vi "_editDialog.vi"(0 "reference":refnum<class "FinalStateNode.lvclass">, 1 "insidePackageNode":bool, 5 "error in (no error)":errorcluster) -> (14 "reference out":refnum<class "FinalStateNode.lvclass">, 15 "changeConnection":T1, 16 "cancel":bool, 19 "error out":errorcluster)   [LabVIEW 2014, in "FinalStateNode.lvclass"]
doc: "Edit Dialog"
uses:
  <resource>/Framework/Providers/Open_GDS/UML/FinalStateNode_class/FinalStateNode.lvclass
  <resource>/Framework/Providers/Open_GDS/UML/AbstractNode_class/private/NodeConnectionStatsType.ctl
  <resource>/Framework/Providers/Open_GDS/UML/ContextHelp/ContextHelp_HelpTexts.ctl
  <resource>/Framework/Providers/Open_GDS/UML/MultiLineString_class/MultiLineString.lvclass
  <resource>/Framework/Providers/Open_GDS/UML/AbstractNode_class/AbstractNode.lvclass
panel:
  in  "OK Button":bool
  in  "Cancel Button":bool
  in  "Help":bool
  in  "connection":bool caption="Connect to System"
  in  "Initial text":string
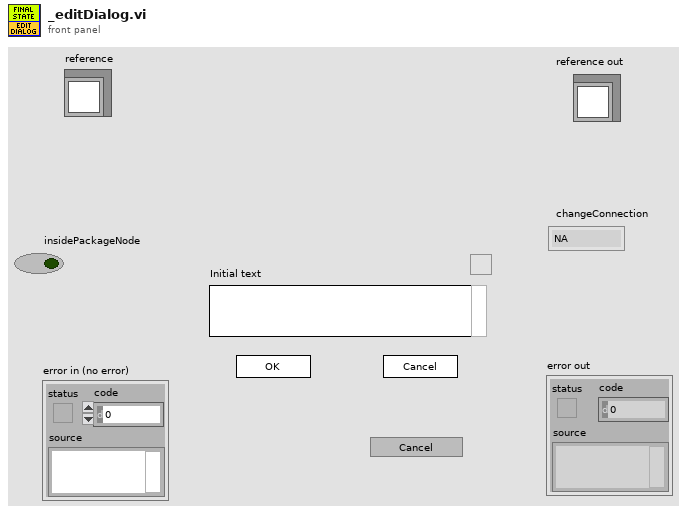
[diagram p1: front panel]
types:
  T1 = typedef "AbstractNode.lvclass/NodeConnectionStatsType.ctl" = enum16{"NA", "Connect", "DisConnect"}
  T2 = typedef "ContextHelp_HelpTexts.ctl" = enum16{"None(Hide)", "Default", "Help", "Welcome", "GettingStarted", "ClassDiagram_Help", "SequenceDiagram_Help", "UseCaseDiagram_Help", "BSelect", "BClass", "BInterface", "BPackage", "BNote", "BDependency", "BInheritance", "BInterfaceImplementation", "BAssociation", "BAggregation", "BCompAggregation", "BNoteConnector", "BObject", "BActionBar", "BCall", "BSystem", "BActor", "BUseCase", "BGeneralization", "BIncludes", "BExtends", "BUseCaseDiagramAssociation", "ClassRelationshipEdge editDialog_Bent Style", "ClassRelationshipEdge editDialog_RelationType", "ClassRelationshipEdge editDialog_Reverse association", "ClassRelationshipEdge editDialog_Start label", "ClassRelationshipEdge editDialog_Middle label", "ClassRelationshipEdge editDialog_End label", "UMLEditor reversedEngineering_Pathes", "ReversedEngineering StateReverseDialog_Help", "ReversedEngineering StateQueuedSettings_Help", "UMLEditor reversedEngineering_AddTopVIs", "UMLEditor reversedEngineering_AddClasses", "UMLEditor reversedEngineering_AddDirs", "UMLEditor reversedEngineering_Recursively", "UMLEditor reversedEngineering_Remove", "UMLEditor reversedEngineering_ClearList", "UMLEditor reversedEngineering_HideSubAss", "UMLEditor reversedEngineering_CreateTypes", "UMLEditor reversedEngineering_OnlyInheritance", "UMLEditor reversedEngineering_CreateApplication", "UMLEditor reversedEngineering_OK", "UMLEditor reversedEngineering_Cancel", "UMLEditor reversedEngineering_Help", "UMLEditor createWizardScriptFile_ScriptfilePath", "UMLEditor createWizardScriptFile_ClassPath", "UMLEditor createWizardScriptFile_Use", "UMLEditor createWizardScriptFile_PrivateDirName", "UMLEditor createWizardScriptFile_DirAppend", "UMLEditor createWizardScriptFile_Separator Character", "UMLEditor createWizardScriptFile_OK", "UMLEditor createWizardScriptFile_Cancel", "UMLEditor createWizardScriptFile_Help", "ClassNode editDialog_Class Name", "InterfaceNode editDialog_Class Name", "ClassNode editDialog_Attribute", "ClassNode editDialog_Methods", "InterfaceNode editDialog_Methods", "ClassNode editDialog_connection", "InterfaceNode editDialog_connection", "ClassNode editDialog_StereoType", "ClassNode editDialog_ShowAttrib", "ClassNode editDialog_ShowMethods", "ClassNode editDialog_ClassPath", "ClassNode editDialog_AddAttribute", "ClassNode editDialog_AddMethod", "InterfaceNode editDialog_AddMethod", "ClassNode AttributeGuide_AttributeName", "ClassNode AttributeGuide_Array?", "ClassNode AttributeGuide_Data Type", "ClassNode AttributeGuide_RefName", "ClassNode AttributeGuide_Preview", "ClassNode AttributeGuide_OK", "ClassNode AttributeGuide_Cancel", "ClassNode MethodGuide_Visibility", "ClassNode MethodGuide_Method Name", "ClassNode MethodGuide_Preview", "ClassNode MethodGuide_OK", "ClassNode MethodGuide_Cancel", "CallNode EditCallProperties_AllButtons", "ObjectNode EditObjectlProperties_AllButtons", "ActorNode EditActorProperties_AllButtons", "UseCaseRelationshipNode EditUseCaselProperties_AllButtons", "UseCaseNode EditUseCaselProperties_AllButtons", "SystemNode EditSystemProperties_AllButtons", "ReversedEngineering UpdateAttributes_AllButtons", "StateNode editDialog_AllButtons", "StateTransition editDialog_AllButtons", "ArrangeNodes Main_Picture", "ArrangeNodes Main_Zoom", "ArrangeNodes Main_Auto Zoom", "ArrangeNodes Main_shorten", "ArrangeNodes Main_Min Length", "ArrangeNodes Main_Max Length", "ArrangeNodes Main_increase", "ArrangeNodes Main_decrease", "ArrangeNodes Main_Shake", "ArrangeNodes Main", "BState", "BInitialState", "BFinalState", "BStateTransition", "StateDiagram_Help", "StateDiagram_PropertiesAllButtons", "ReversedEngineering StateReverseDialog_ClearStates", "ReversedEngineering StateReverseDialog_UseQueuedStateMachines", "ReversedEngineering StateReverseDialog_QueuedSettings", "ReversedEngineering StateReverseDialog_SearchForVIs", "ReversedEngineering StateReverseDialog_SearchCriteria", "OptionsDialog_ClassBasePath", "OptionsDialog_VIPath", "OptionsDialog_ApplicationPath", "OptionsDialog_WizDir", "OptionsDialog_IniFilePath", "OptionsDialog_DefineColors", "OptionsDialog_Help", "OptionsDialog_CreateTypes", "ClassRelationshipEdge editDialog_SplitWire"}
  T3 = typedef "FinalStateNode.lvclass/ObjectAttributes.ctl" = cluster{"name":refnum<class "MultiLineString.lvclass">, "DEFAULT_WIDTH":i32, "DEFAULT_HEIGHT":i32}
  T4 = typedef "AbstractNode.lvclass/ObjectAttributes.ctl" = cluster{"parent":refnum<class "AbstractNode.lvclass">, "children":refnum<class "AbstractNode.lvclass">[], "Hidden":bool}
  T5 = typedef "ContextHelp_ShowType.ctl" = cluster{"Header":string, "Picture":picture, "Text":string}
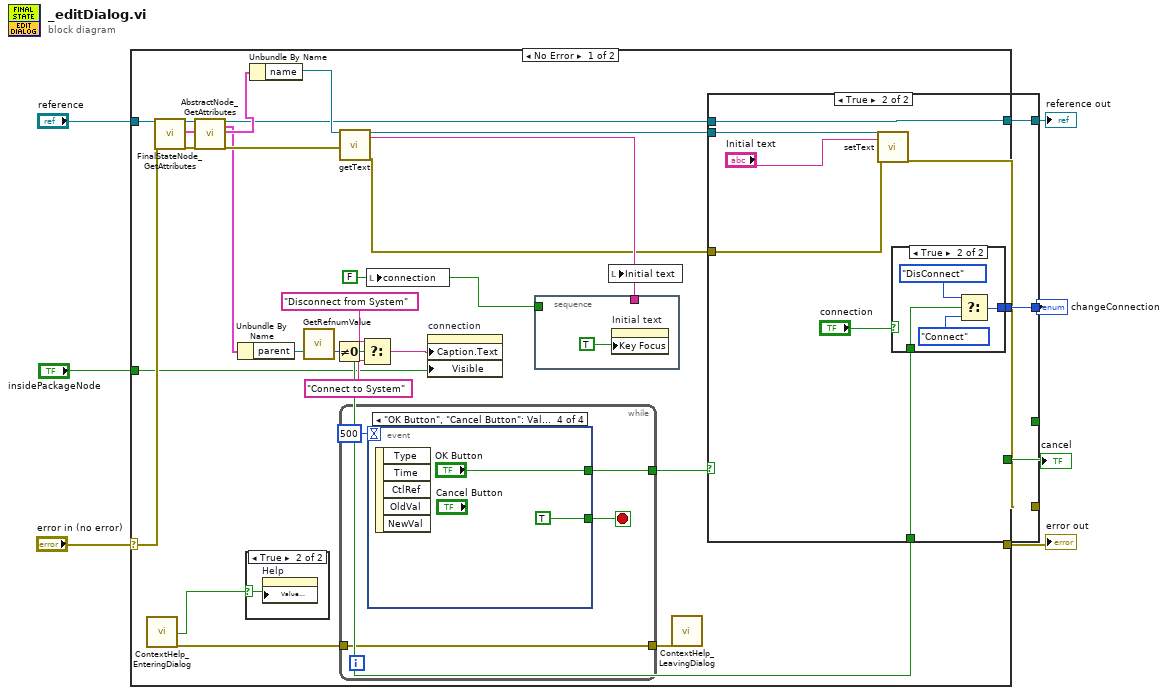
[diagram p0: block diagram]
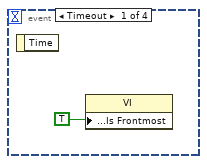
[diagram p3: hidden frame]
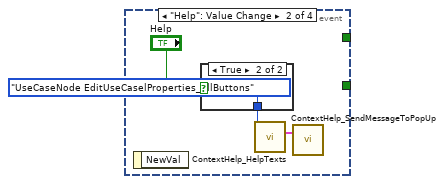
[diagram p4: hidden frame]
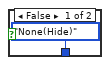
[diagram p5: hidden frame]
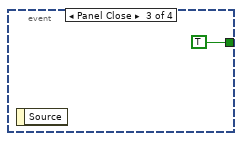
[diagram p6: hidden frame]
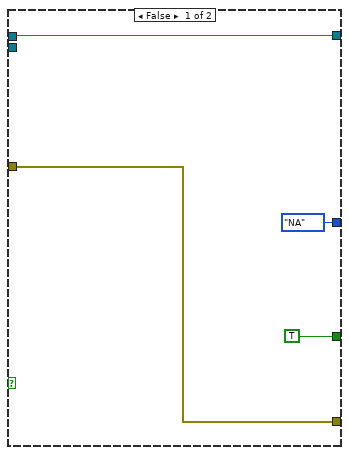
[diagram p7: hidden frame]
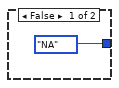
[diagram p8: hidden frame]
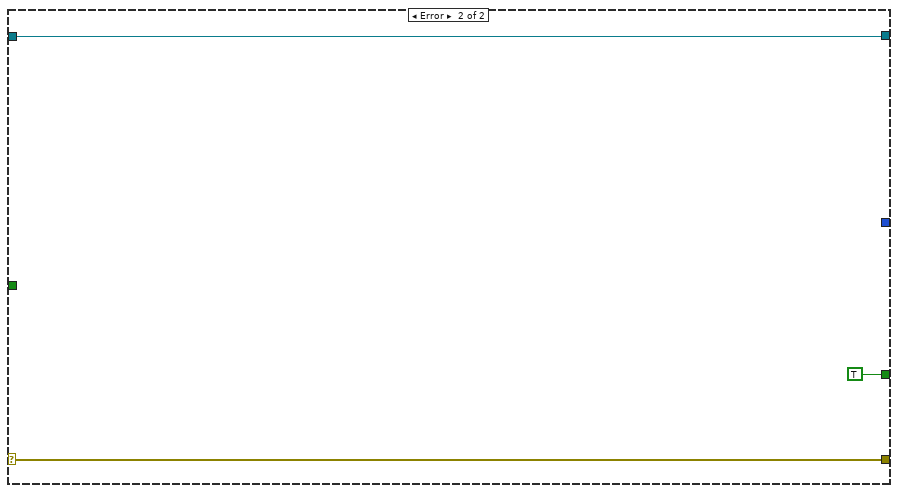
[diagram p9: hidden frame]
diagram:
  n1 = case shown="No Error" "error in (no error)" {
    selector: "error in (no error)" -> [w32 w69]
    tunnel: "reference" -> [w33 w70]
    tunnel: [w35 w69] -> w5
    tunnel: [w34 w70] -> w4
    tunnel: [w28 _] -> w3
    tunnel: "insidePackageNode" -> [w23 _]
    tunnel: [w21 TRUE ("Key Focus")] -> w1
    frame No Error {
      w22 = FALSE ("connection")
      n2 = call <resource>:"ContextHelp_EnteringDialog.vi"() -> ("HelpStatus"=w16:bool, "error out"=w18:errorcluster)  [unwired: 3 in, 15 out]
      n3 = call <resource>:"FinalStateNode_GetAttributes.vi"("reference in"=w33, "error in (no error)"=w32) -> ("reference out"=w12:refnum<class "FinalStateNode.lvclass">, "Data"=w13:T3, "error out"=w11:errorcluster)  [unwired: 1 in, 14 out]
      n4 = call <resource>:"AbstractNode_GetAttributes.vi"("reference in"=w12, "error in (no error)"=w11) -> ("reference out"=w9:refnum<class "FinalStateNode.lvclass">, "Data"=w8:T4, "error out"=w10:errorcluster)  [unwired: 14 in, 1 out]
      n5 = Unbundle By Name(w8) -> ("parent"=w15:refnum<class "AbstractNode.lvclass">)
      n6 = case shown="True" w16 {
        selector: w16 -> [_ w36]
        frame False {
        }
        frame True {
          n7 = property on="Help" class="Bool (strict)"("Value (Signaling)"=w36) -> ()  [unwired: 2 in, 2 out]
        }
      }
      n8 = Unbundle By Name(w13) -> ("name"=w29:refnum<class "MultiLineString.lvclass">)
      n9 = call <resource>:"GetRefnumValue.vi"("reference"=w15) -> ("RefNum"=w14:i32)  [unwired: 17 in, 1 out]
      n10 = Not Equal To 0?(x=w14) -> (x != 0?=w27:bool)
      n11 = call-dynamic "getText.vi"("reference"=w29, "error in (no error)"=w10) -> ("reference out"=w31:refnum<class "MultiLineString.lvclass">, "text"=w30:string, "error out"=w20:errorcluster)  [unwired: 15 in]
      n12 = while {
        tunnel: [w40] -> w17
        tunnel: [w38] -> w19
        tunnel: w18 -> [w38]
        stop <- w39 stop-if-true
        n13 = event shown="[3] \"OK Button\", \"Cancel Button\": Value Change" {
          selector: _ -> [_ _ _ _]
          dyn-events: _ -> [_ _ _ _]
          timeout: 500 -> [_ _ _ _]
          tunnel: [_ _ _ "OK Button"] -> w40
          tunnel: [_ _ TRUE TRUE] -> w39
          event Timeout {
            n14 = event-data() -> ()  [unwired: 2 out]
            n15 = property class="VI"("Front Panel Window:Is Frontmost"=TRUE) -> ()  [unwired: 2 in, 2 out]
          }
          event "Help": Value Change {
            n16 = event-data() -> ()  [unwired: 2 out]
            n17 = case shown="True" "Help" {
              tunnel: [ContextHelp_HelpTexts."None(Hide)" ("HelpText") ContextHelp_HelpTexts."UseCaseNode EditUseCaselProperties_AllButtons" ("HelpText")] -> w43
              frame False {
              }
              frame True {
              }
            }
            n18 = call <resource>:"ContextHelp_HelpTexts.vi"("HelpText (enum or string)"=w43) -> ("HelpOut"=w44:T5)  [unwired: 18 out]
            n19 = call <resource>:"ContextHelp_SendMessageToPopUp.vi"("PopUpMessage"=w44) -> ()  [unwired: 2 in, 17 out]
          }
          event Panel Close {
            n20 = event-data() -> ()  [unwired: 2 out]
          }
          event "OK Button", "Cancel Button": Value Change {
            n21 = event-data() -> ()  [unwired: 6 out]
          }
        }
      }
      n22 = Select(t="Disconnect from System", s=w27, f="Connect to System") -> (s? t:f=w26:string)
      n23 = local write "connection"(w22) -> ()
      n24 = property on="connection" class="Bool (strict)"("Caption.Text"=w26, "Visible"=w23) -> ()  [unwired: 2 in, 2 out]
      n25 = stacked-sequence {
        tunnel: w30 -> [_]
        tunnel: w22 -> [_]
        frame #0 {
          n26 = property on="Initial text" class="Str"("Key Focus"=TRUE) -> ()  [unwired: 2 in, 2 out]
        }
      }
      n27 = local write "Initial text"(w30) -> ()
      n28 = call <resource>:"ContextHelp_LeavingDialog.vi"("error in (no error)"=w19) -> ()  [unwired: 2 in, 17 out]
      n29 = case shown="True" w17 {
        tunnel: [w52 w58] -> w35
        tunnel: [w53 w59] -> w34
        tunnel: w9 -> [w53 w59]
        tunnel: w31 -> [_ w61]
        tunnel: w20 -> [w52 w54]
        tunnel: [enum16{"NA", "Connect", "DisConnect"}."NA" ("changeConnection") w56] -> w28
        tunnel: w27 -> [_ w55]
        tunnel: [TRUE ("Key Focus") _] -> w21
        frame False {
        }
        frame True {
          n30 = call-dynamic "setText.vi"("reference"=w61, "text"="Initial text", "error in (no error)"=w54) -> ("error out"=w58:errorcluster)  [unwired: 15 in, 1 out]
          n31 = case shown="True" "connection" {
            tunnel: [enum16{"NA", "Connect", "DisConnect"}."NA" ("changeConnection") w65] -> w56
            tunnel: w55 -> [_ w66]
            frame False {
            }
            frame True {
              n32 = Select(t=enum16{"NA", "Connect", "DisConnect"}."DisConnect" ("changeConnection"), s=w66, f=enum16{"NA", "Connect", "DisConnect"}."Connect" ("changeConnection")) -> (s? t:f=w65:enum16{"NA", "Connect", "DisConnect"})
            }
          }
        }
      }
    }
    frame Error {
    }
  }
  "reference out" <- w4
  "error out" <- w5
  "changeConnection" <- w3
  "cancel" <- w1
